vi "SQL.INIFile.vi"(4 "error in (no error)":errorcluster caption="错误输入（无错误）", 7 "Folder Path":path caption="文件夹路径") -> (0 "错误输出":errorcluster)   [LabVIEW 2012, in "Lib_UEL.ATE.lvlib" / "Lib_SQL.lvlib"]
uses:
  Lib_SQL.lvlib
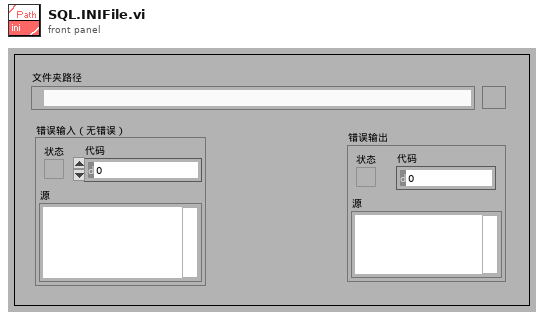
[diagram p1: front panel]
types:
  T1 = enum16{"open", "replace", "create", "open or create", "replace or create", "replace or create with confirmation"}
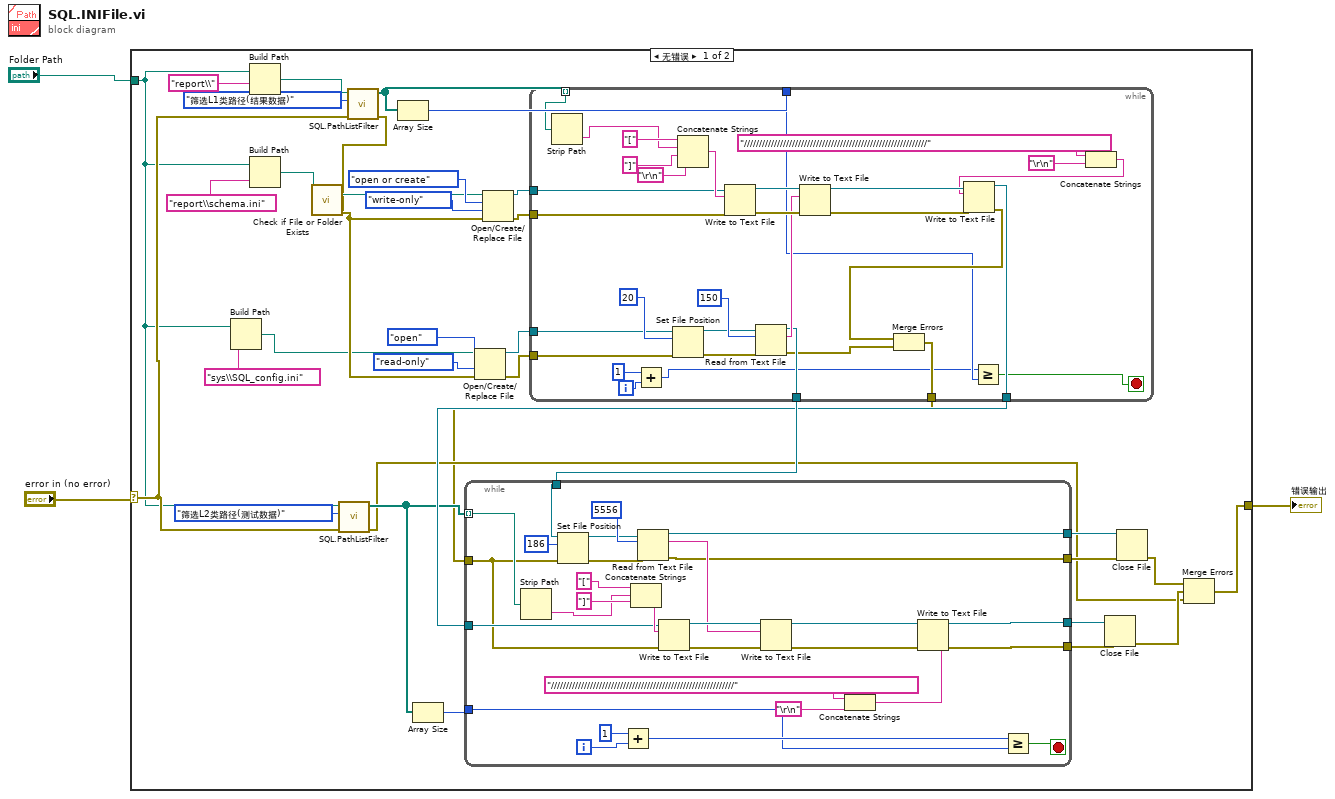
[diagram p0: block diagram]
diagram:
  n1 = case shown="无错误" "error in (no error)" {
    selector: "error in (no error)" -> [w23 w101]
    tunnel: [w31 w101] -> w2
    tunnel: "Folder Path" -> [w6 _]
    frame No Error {
      n2 = Build Path(base path=w6, name or relative path="sys\\SQL_config.ini" ("名称或相对路径")) -> (appended path=w18:path)
      n3 = Build Path(base path=w6, name or relative path="report\\" ("名称或相对路径")) -> (appended path=w5:path)
      n4 = Build Path(base path=w6, name or relative path="report\\schema.ini" ("名称或相对路径")) -> (appended path=w13:path)
      n5 = call "SQL.PathListFilter.vi"("错误输入"=w23, "CMD"=enum16{"筛选L1类路径(结果数据)", "筛选L2类路径(测试数据)"}."筛选L2类路径(测试数据)", "Folder Path"=w6) -> ("错误输出"=w24:errorcluster, "PathList_Output"=w25:path[])  [unwired: 7 in]
      n6 = call "SQL.PathListFilter.vi"("错误输入"=w23, "CMD"=enum16{"筛选L1类路径(结果数据)", "筛选L2类路径(测试数据)"}."筛选L1类路径(结果数据)", "Folder Path"=w5) -> ("错误输出"=w11:errorcluster, "PathList_Output"=w29:path[])  [unwired: 7 in]
      n7 = call <vilib>:"Check if File or Folder Exists.vi"("error in (no error)"=w11, "path"=w13) -> ("error out"=w21:errorcluster, "dup path"=w14:path)  [unwired: 7 in, 1 out]
      n8 = Array Size(array=w29) -> (size(s)=w28:i32)
      n9 = Array Size(array=w25) -> (size(s)=w26:i32)
      n10 = Open/Create/Replace File(file path (use dialog)=w18, error in=w21, operation (0:open)=T1."open" ("运行（0:打开）"), access (0:read/write)=enum16{"read/write", "read-only", "write-only"}."read-only" ("访问（0:读取/写入）")) -> (refnum out=w8:refnum<file>, error out=w7:errorcluster)  [unwired: 2 in, 1 out]
      n11 = Open/Create/Replace File(file path (use dialog)=w14, error in=w21, operation (0:open)=T1."open or create" ("运行（0:打开）"), access (0:read/write)=enum16{"read/write", "read-only", "write-only"}."write-only" ("访问（0:读取/写入）")) -> (refnum out=w10:refnum<file>, error out=w9:errorcluster)  [unwired: 2 in, 1 out]
      n12 = while {
        tunnel: [w62] -> w39
        tunnel: [w60] -> w38
        tunnel: [w51] -> w22
        tunnel: w29 -> [w45] mode=indexing
        tunnel: w28 -> [w48]
        tunnel: w10 -> [w43]
        tunnel: w9 -> [w42]
        tunnel: w8 -> [w41]
        tunnel: w7 -> [w40]
        i -> [w49]
        stop <- w46 stop-if-true
        n13 = Strip Path(path=w45) -> (name=w44:string)  [unwired: 1 out]
        n14 = Add(x=1, y=w49) -> (x+y=w47:i32)
        n15 = Set File Position(offset (in bytes) (0)=i64 20 ("偏移量（字节）（0）"), refnum=w41, error in=w40) -> (refnum out=w67:refnum<file>, error out=w58:errorcluster)  [unwired: 1 in]
        n16 = Concatenate Strings("[", w44, "]", "\r\n") -> (w69:string)
        n17 = Write to Text File(file (use dialog)=w43, text=w69, error in=w42) -> (refnum out=w63:refnum<file>, error out=w66:errorcluster)  [unwired: 1 in, 1 out]
        n18 = Read from Text File(file (use dialog)=w67, count=150 ("计数"), error in=w58) -> (refnum out=w62:refnum<file>, text=w65:string, error out=w53:errorcluster)  [unwired: 1 in, 1 out]
        n19 = Write to Text File(file (use dialog)=w63, text=w65, error in=w66) -> (refnum out=w61:refnum<file>, error out=w57:errorcluster)  [unwired: 1 in, 1 out]
        n20 = Greater Or Equal?(x=w47, y=w48) -> (x >= y?=w46:bool)
        n21 = Concatenate Strings("/////////////////////////////////////////////////////////////" ("文本"), "\r\n") -> (w56:string)
        n22 = Write to Text File(file (use dialog)=w61, text=w56, error in=w57) -> (refnum out=w60:refnum<file>, error out=w52:errorcluster)  [unwired: 1 in, 1 out]
        n23 = Merge Errors(w52, w53) -> (w51:errorcluster)
      }
      n24 = while {
        tunnel: w39 -> [w97]
        tunnel: w38 -> [w83]
        tunnel: w22 -> [w72]
        tunnel: [w79] -> w37
        tunnel: [w78] -> w36
        tunnel: [w77] -> w35
        tunnel: [w76] -> w34
        tunnel: w26 -> [w74]
        tunnel: w25 -> [w73] mode=indexing
        i -> [w89]
        stop <- w86 stop-if-true
        n25 = Strip Path(path=w73) -> (name=w91:string)  [unwired: 1 out]
        n26 = Set File Position(offset (in bytes) (0)=i64 186 ("偏移量（字节）（0）"), refnum=w97, error in=w72) -> (refnum out=w98:refnum<file>, error out=w80:errorcluster)  [unwired: 1 in]
        n27 = Add(x=1, y=w89) -> (x+y=w87:i32)
        n28 = Concatenate Strings("[", w91, "]") -> (w94:string)
        n29 = Read from Text File(file (use dialog)=w98, count=5556 ("计数"), error in=w80) -> (refnum out=w79:refnum<file>, text=w90:string, error out=w77:errorcluster)  [unwired: 1 in, 1 out]
        n30 = Write to Text File(file (use dialog)=w83, text=w94, error in=w72) -> (refnum out=w96:refnum<file>, error out=w95:errorcluster)  [unwired: 1 in, 1 out]
        n31 = Write to Text File(file (use dialog)=w96, text=w90, error in=w95) -> (refnum out=w85:refnum<file>, error out=w84:errorcluster)  [unwired: 1 in, 1 out]
        n32 = Concatenate Strings("/////////////////////////////////////////////////////////////" ("文本"), "\r\n") -> (w81:string)
        n33 = Write to Text File(file (use dialog)=w85, text=w81, error in=w84) -> (refnum out=w78:refnum<file>, error out=w76:errorcluster)  [unwired: 1 in, 1 out]
        n34 = Greater Or Equal?(x=w87, y=w74) -> (x >= y?=w86:bool)
      }
      n35 = Close File(refnum=w36, error in=w34) -> (error out=w32:errorcluster)  [unwired: 1 out]
      n36 = Close File(refnum=w37, error in=w35) -> (error out=w33:errorcluster)  [unwired: 1 out]
      n37 = Merge Errors(w33, w32, w24) -> (w31:errorcluster)
    }
    frame Error {
    }
  }
  "错误输出" <- w2
